vi "PhasePID.vi"(4 "Kd/Tau":fxp<+/-,32,4>, 5 "Ki*Tau":fxp<+/-,32,4>, 6 "Kp":fxp<+/-,32,4>, 7 "Reset":bool, 8 "input valid":bool=TRUE, 9 "Fi_delta":fxp<+/-,32,4>, 10 "Fi_start":fxp<+/-,32,4>, 11 "Data in":fxp<+/-,16,14>[](array[numeric])=[0.0, 0.0, 0.0, 0.0]) -> (0 "output valid":bool, 2 "Fi_korr":fxp<+/-,32,4>, 3 "Fi_korr PID":fxp<+/-,32,4>)   [LabVIEW 2013]
uses:
  <vilib>/rvi/FXPMathLib/FxpSub/XNode/nifxpmath_Sub.xnode
  <vilib>/rvi/FXPMathLib/FxpAdd/XNode/nifxpmath_Add.xnode
  <vilib>/rvi/FXPMathLib/FxpMul/XNode/nifxpmath_Multiplier.xnode
  <vilib>/rvi/FXPMathLib/sim/FxpSim.dll
panel:
  # "2*Pi*Fc*T_delay"
  # "2*Pi*Fc*delta_fi_increase"
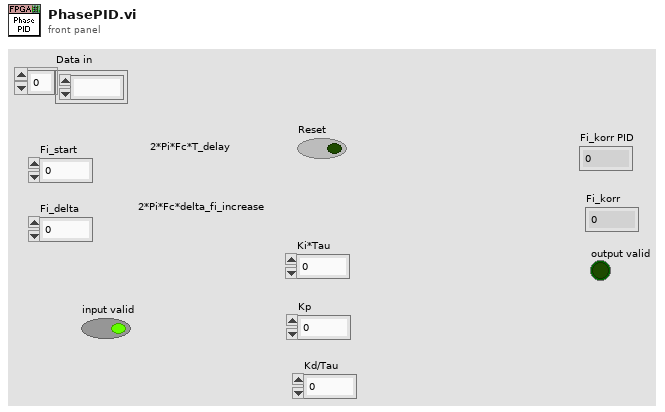
[diagram p1: front panel]
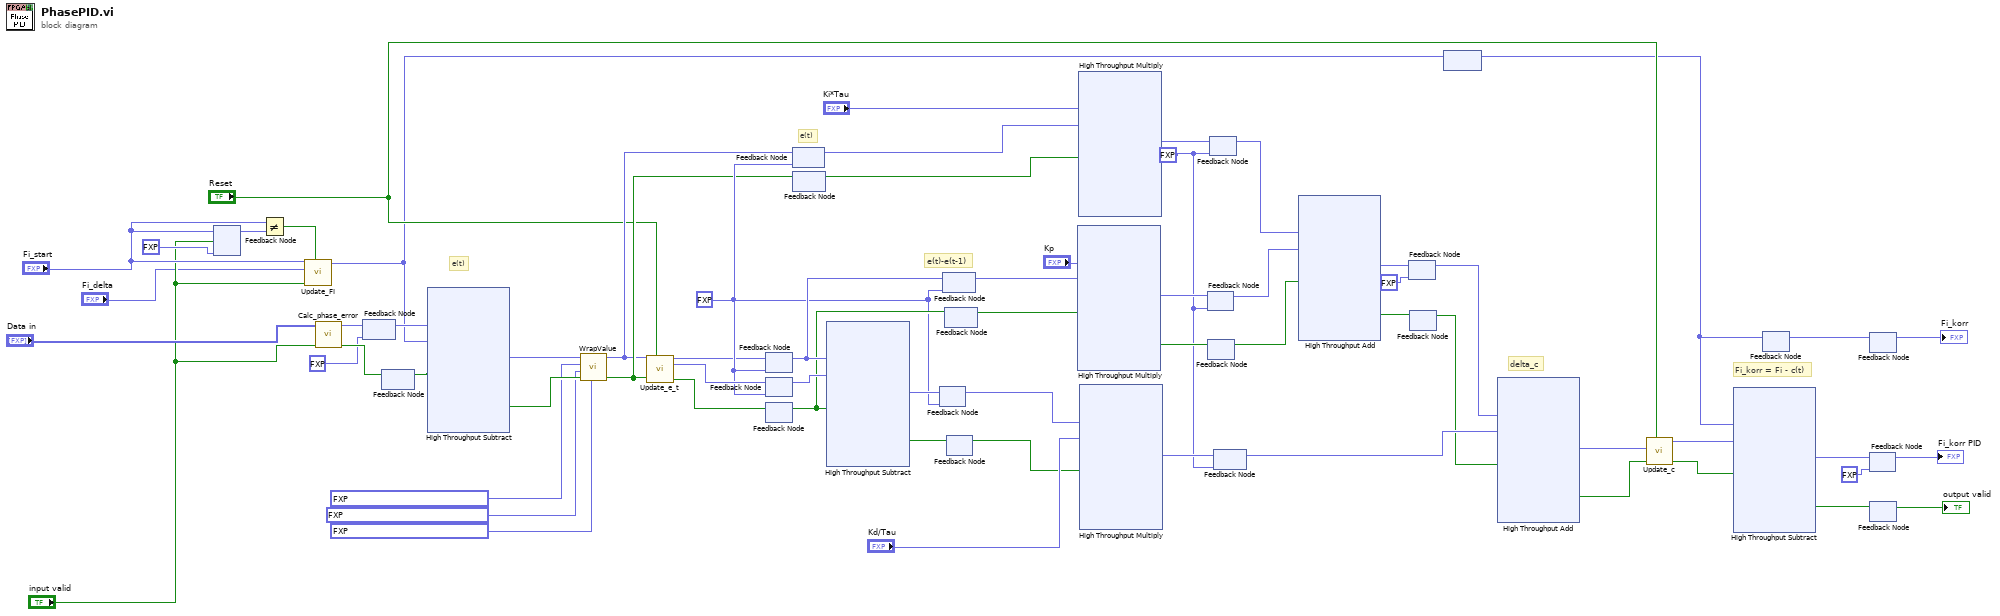
[diagram p0: block diagram]
diagram:
  w25 = fxp<+/-,32,4> 0.0 ("x*y")
  w24 = fxp<+/-,32,4> 0.0 ("x*y")
  # "Fi_korr = Fi - c(t)"
  # "delta_c"
  # "e(t)-e(t-1)"
  # "e(t)"
  # "e(t)"
  n1 = feedback #1(fxp<+/-,32,4> -1.0 ("Fi_start")) -> (w7:fxp<+/-,32,4>)
  n2 = feedback-in #1("Fi_start", "input valid") -> ()
  n3 = Not Equal?(x="Fi_start", y=w7) -> (x != y?=w4:bool)
  n4 = call "Update_FI.vi"("Reset"=w4, "input valid"="input valid", "Fi_delta"="Fi_delta", "Fi_start"="Fi_start") -> ("Fi out"=w3:fxp<+/-,32,4>)  [unwired: 6 in, 1 out]
  n5 = call "Calc_phase_error.vi"("input valid"="input valid", "Data in"="Data in") -> ("output valid"=w32:bool, "Phase error"=w31:fxp<+/-,32,4>)  [unwired: 8 in]
  n6 = feedback #2(fxp<+/-,32,4> 0.0 ("x*y")) -> (w33:fxp<+/-,32,4>)
  n7 = feedback-in #2(w31) -> ()
  n8 = feedback #3() -> (w64:bool)  [unwired: 1 in]
  n9 = feedback-in #3(w32) -> ()
  n10 = xnode "High Throughput Subtract"("x"=w33, "y"=w3, "input valid"=w64) -> ("x-y"=w54:fxp<+/-,32,4>, "output valid"=w53:bool)  [unwired: 1 in, 1 out]
  n11 = call "WrapValue.vi"("wrap_range"=fxp<+/-,32,4> 6.2831853069365025 ("wrap_max"), "Input valid"=w53, "wrap_min"=fxp<+/-,32,4> -3.1415926553308964 ("wrap_max"), "wrap_max"=fxp<+/-,32,4> 3.1415926553308964, "x_in"=w54) -> ("output valid"=w19:bool, "x_out"=w18:fxp<+/-,32,4>)  [unwired: 5 in]
  n12 = call "Update_e_t.vi"("Reset"="Reset", "input valid"=w19, "e(t)"=w18) -> ("output valid"=w21:bool, "e(t-1)-e(t-2)"=w63:fxp<+/-,32,4>, "e(t)-e(t-1)"=w20:fxp<+/-,32,4>)  [unwired: 6 in]
  n13 = feedback #4(w25) -> (w37:fxp<+/-,32,4>)
  n14 = feedback-in #4(w20) -> ()
  n15 = feedback #5(w25) -> (w62:fxp<+/-,32,4>)
  n16 = feedback-in #5(w63) -> ()
  n17 = feedback #6() -> (w35:bool)  [unwired: 1 in]
  n18 = feedback-in #6(w21) -> ()
  n19 = feedback #7(w25) -> (w56:fxp<+/-,32,4>)
  n20 = feedback-in #7(w18) -> ()
  n21 = feedback #8() -> (w48:bool)  [unwired: 1 in]
  n22 = feedback-in #8(w19) -> ()
  n23 = xnode "High Throughput Subtract"("x"=w37, "y"=w62, "input valid"=w35) -> ("x-y"=w60:fxp<+/-,32,4>, "output valid"=w59:bool)  [unwired: 1 in, 1 out]
  n24 = feedback #9(w25) -> (w58:fxp<+/-,32,4>)
  n25 = feedback-in #9(w60) -> ()
  n26 = feedback #10(w25) -> (w36:fxp<+/-,32,4>)
  n27 = feedback-in #10(w37) -> ()
  n28 = feedback #11() -> (w34:bool)  [unwired: 1 in]
  n29 = feedback-in #11(w35) -> ()
  n30 = feedback #12() -> (w49:bool)  [unwired: 1 in]
  n31 = feedback-in #12(w59) -> ()
  n32 = xnode ("High Throughput Multiply")("x"="Kp", "y"=w36, "input valid"=w34) -> ("x*y"=w45:fxp<+/-,32,4>, "output valid"=w44:bool)  [unwired: 1 in, 1 out]
  n33 = xnode ("High Throughput Multiply")("x"="Ki*Tau", "y"=w56, "input valid"=w48) -> ("x*y"=w47:fxp<+/-,32,4>)  [unwired: 1 in, 2 out]
  n34 = xnode ("High Throughput Multiply")("x"=w58, "y"="Kd/Tau", "input valid"=w49) -> ("x*y"=w43:fxp<+/-,32,4>)  [unwired: 1 in, 2 out]
  n35 = feedback #13(w24) -> (w29:fxp<+/-,32,4>)
  n36 = feedback-in #13(w45) -> ()
  n37 = feedback #14() -> (w30:bool)  [unwired: 1 in]
  n38 = feedback-in #14(w44) -> ()
  n39 = feedback #15(w24) -> (w46:fxp<+/-,32,4>)
  n40 = feedback-in #15(w47) -> ()
  n41 = feedback #16(w24) -> (w42:fxp<+/-,32,4>)
  n42 = feedback-in #16(w43) -> ()
  n43 = xnode "High Throughput Add"("x"=w46, "y"=w29, "input valid"=w30) -> ("x+y"=w41:fxp<+/-,32,4>, "output valid"=w40:bool)  [unwired: 1 in, 1 out]
  n44 = feedback #17(fxp<+/-,32,4> 0.0 ("x*y")) -> (w39:fxp<+/-,32,4>)
  n45 = feedback-in #17(w41) -> ()
  n46 = feedback #18() -> (w38:bool)  [unwired: 1 in]
  n47 = feedback-in #18(w40) -> ()
  n48 = feedback #19() -> (w10:fxp<+/-,32,4>)  [unwired: 1 in]
  n49 = feedback-in #19(w3) -> ()
  n50 = xnode "High Throughput Add"("x"=w39, "y"=w42, "input valid"=w38) -> ("x+y"=w26:fxp<+/-,32,4>, "output valid"=w27:bool)  [unwired: 1 in, 1 out]
  n51 = call "Update_c.vi"("Reset"="Reset", "input valid"=w27, "delta_c"=w26) -> ("output valid"=w28:bool, "c out"=w15:fxp<+/-,32,4>)  [unwired: 7 in]
  n52 = xnode "High Throughput Subtract"("x"=w10, "y"=w15, "input valid"=w28) -> ("x-y"=w12:fxp<+/-,32,4>, "output valid"=w11:bool)  [unwired: 1 in, 1 out]
  n53 = feedback #20() -> (w9:fxp<+/-,32,4>)  [unwired: 1 in]
  n54 = feedback-in #20(w10) -> ()
  n55 = feedback #21(fxp<+/-,32,4> 0.0 ("x*y")) -> (→"Fi_korr PID":fxp<+/-,32,4>)
  n56 = feedback-in #21(w12) -> ()
  n57 = feedback #22() -> (→"Fi_korr":fxp<+/-,32,4>)  [unwired: 1 in]
  n58 = feedback-in #22(w9) -> ()
  n59 = feedback #23() -> (→"output valid":bool)  [unwired: 1 in]
  n60 = feedback-in #23(w11) -> ()
